vi "GetLocals.vi"(6 "error in":errorcluster, 9 "Diagram in":refnum<class "Diagram.lvclass">) -> (0 "error out":errorcluster, 3 "Diagram out":refnum<class "Diagram.lvclass">, 4 "locals":i32[](array[numeric]))   [LabVIEW 2014, in "Diagram.lvclass"]
uses:
  Diagram.lvclass
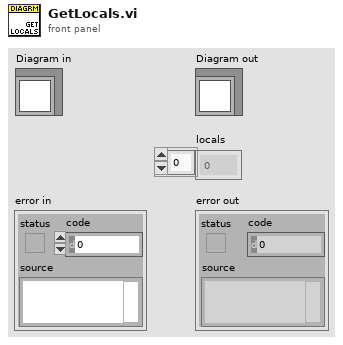
[diagram p1: front panel]
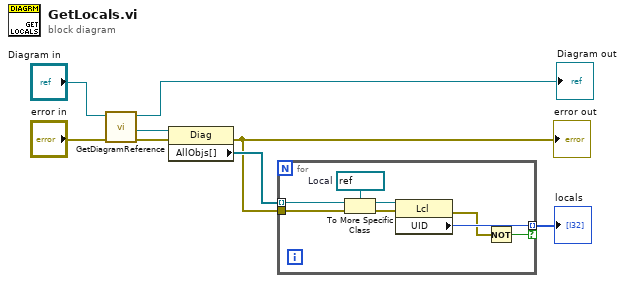
[diagram p0: block diagram]
diagram:
  n1 = call "GetDiagramReference.vi"("error in"="error in", "Diagram in"="Diagram in") -> ("error out"=w5:errorcluster, "reference out"=w4:refnum<vi>, "Diagram out"=→"Diagram out":refnum<class "Diagram.lvclass">)  [unwired: 5 in]
  n2 = property class="Diag"(reference=w4, error in=w5) -> (error out=w1:errorcluster, "AllObjs[]"=w3:refnum<vi>[])  [unwired: 1 out]
  "error out" <- w1
  n3 = for {
    tunnel: w3 -> [w16] mode=indexing
    tunnel: w1 -> [w15]
    tunnel: [w11] -> w2 mode=indexing if=w9
    w14 = refnum<vi> refnum  # Local
    n4 = To More Specific Class(target class=w14, reference=w16, error in=w15) -> (specific class reference=w13:refnum<vi>, error out=w12:errorcluster)
    n5 = property class="Lcl"(reference=w13, error in=w12) -> (error out=w10:errorcluster, "UID"=w11:i32)  [unwired: 1 out]
    n6 = Not(x=w10) -> (.not. x?=w9:bool)
  }
  "locals" <- w2
